vi "Set Temperature.vi"(8 "error in (no error)":errorcluster, 11 "Cooler in":refnum<class "Cooler.lvclass">) -> (0 "error out":errorcluster, 3 "Cooler out":refnum<class "Cooler.lvclass">)   [LabVIEW 2018, in "Cooler.lvclass"]
uses:
  Cooler.lvclass
  Cooler.lvclass/Cooler.ctl
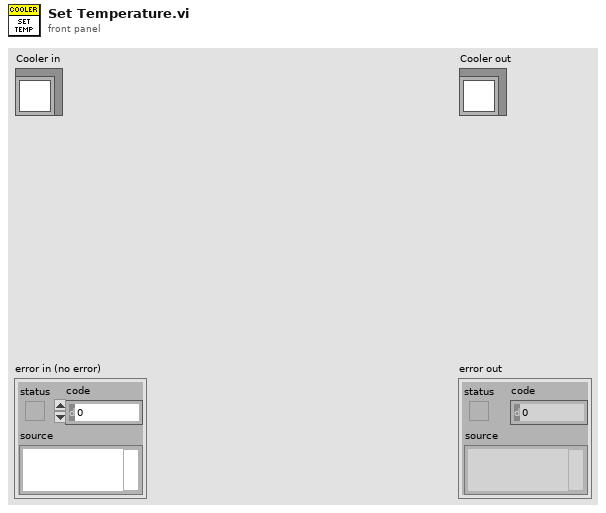
[diagram p1: front panel]
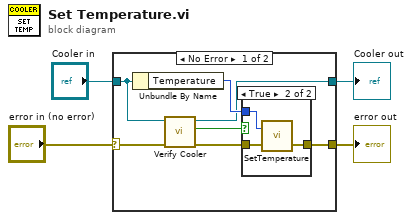
[diagram p0: block diagram]
diagram:
  n1 = case shown="No Error" "error in (no error)" {
    selector: "error in (no error)" -> [w8 w17]
    tunnel: [w11 w17] -> w2
    tunnel: [w6 w16] -> w3
    tunnel: "Cooler in" -> [w7 w16]
    frame No Error {
      n2 = Unbundle By Name(w7) -> ("Temperature"=w10:i32)
      n3 = call "Verify Cooler.vi"("error in (no error)"=w8, "Cooler in"=w7) -> ("error out"=w9:errorcluster, "coolerStatus"=w5:bool, "Cooler out"=w6:refnum<class "Cooler.lvclass">)  [unwired: 7 in]
      n4 = case shown="True" w5 {
        tunnel: [w12 w15] -> w11
        tunnel: w10 -> [_ w14]
        tunnel: w9 -> [w12 w13]
        frame False {
        }
        frame True {
          n5 = call <userlib>:"SetTemperature.vi"("error in (no error)"=w13, "temperature"=w14) -> ("error out"=w15:errorcluster)  [unwired: 1 out]
        }
      }
    }
    frame Error {
    }
  }
  "error out" <- w2
  "Cooler out" <- w3
